vi "FPGA_Write.vi"(5 "Espera acceso USB":u32=10, 6 "error in":errorcluster, 7 "Bytes de escritura":u8[](array[numeric]), 8 "Dirección base":u8, 9 "ftHandle_in":u32) -> (0 "error out":errorcluster, 1 "lpBytesWritten":u32, 2 "status":u32, 3 "ftHandle_out":u32)   [LabVIEW 2019]
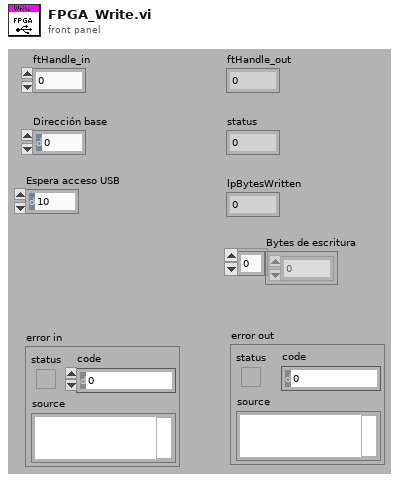
[diagram p1: front panel]
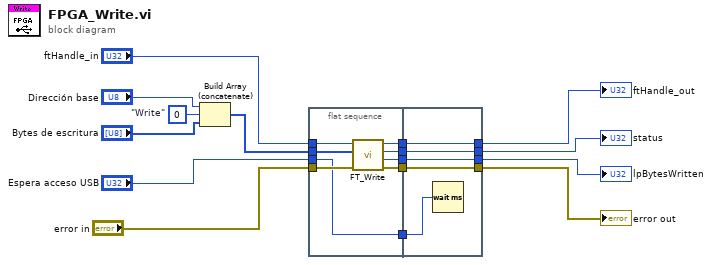
[diagram p0: block diagram]
diagram:
  w8 = u8 0  # "Write"
  n1 = Build Array (concatenate)("Dirección base", w8, "Bytes de escritura") -> (w7:u8[])
  n2 = flat-sequence {
    tunnel: "error in" -> [w24]
    tunnel: "ftHandle_in" -> [w20]
    tunnel: w7 -> [w19]
    tunnel: [w23] -> w6
    tunnel: [w18] -> w5
    tunnel: [w22] -> w4
    tunnel: [w21] -> w3
    tunnel: [w17] -> w2
    tunnel: "Espera acceso USB" -> [w17]
    tunnel: [w26] -> w11
    tunnel: [w27] -> w12
    tunnel: [w28] -> w13
    tunnel: [w29] -> w14
    tunnel: w6 -> [w29]
    tunnel: w5 -> [w28]
    tunnel: w4 -> [w27]
    tunnel: w3 -> [w26]
    tunnel: w2 -> [w25]
    frame #0 {
      n3 = call "FT_Write.vi"("error in (no error)"=w24, "lpBuffer"=w19, "ftHandle_in"=w20) -> ("error out"=w22:errorcluster, "lpBytesWritten"=w23:u32, "status"=w18:u32, "ftHandle_out"=w21:u32)  [unwired: 1 in, 4 out]
    }
    frame #1 {
      n4 = Wait (ms)(milliseconds to wait=w25) -> ()  [unwired: 1 out]
    }
  }
  "lpBytesWritten" <- w14
  "status" <- w13
  "error out" <- w12
  "ftHandle_out" <- w11
